vi "FPGA Main.vi"() -> ()   [LabVIEW 2017]
uses:
  Controls/Logging Settings FPGA.ctl
  Controls/Manual Control FPGA.ctl
  <vilib>/rvi/eio/common/nirviEmuTemplateMethod_errors.vi
  <vilib>/rvi/Emulation/niFpgaGetClockAttributes.vi
  <vilib>/rvi/Emulation/niFpgaSctlEmulationGetInTimedLoop.vi
  <vilib>/rvi/Emulation/niFpgaEmulationReportErrorSimple.vi
  <vilib>/rvi/Emulation/niFpgaProcessEmulError.vi
  <vilib>/rvi/interface/RandomDataEmulation/niFpgaRandomDataHandleErrors.vi
  <vilib>/rvi/Emulation/niFpgaCriticalErrorInLSC.vi
  <vilib>/eio/EIONode/EIONode.xnode
  <vilib>/rvi/DataTransferAndStorage/Container/XNode/niFpgaContainer.xnode
  <vilib>/rvi/interface/RandomDataEmulation/nirviRandomDataFpgaReadWriteTemplate.vi
panel:
  out "Emergency Triggered":bool
  in  "Emergency Normally Open/Closed":bool
  in  "Actuator Settings":T1 {"Emergency State" items=["Closed", "Open"]; "Output Port" items=["DIDO/DO0", "DIDO/DO1", "DIDO/DO2", "DIDO/DO3", "DIDO/DO4", "DIDO/DO5", "DIDO/DO6", "DIDO/DO7", "DIDO/DO8", "DIDO/DO9", "DIDO/DO10", "DIDO/DO11", "DIDO/DO12", "DIDO/DO13", "DIDO/DO14", "DIDO/DO15", "PWM/DO0", "PWM/DO1", "PWM/DO2", "PWM/DO3", "PWM/DO4", "PWM/DO5", "PWM/DO6", "PWM/DO7"]; "Unpowered State" items=["Closed", "Opened"]}
  in  "Logging Settings":T2
  out "LC FIFO Timed Out":bool
  out "PS FIFO Timed Out":bool
  in  "Poll Rate":u32
  in  "Logging?":bool
  out "TC FIFO Timed Out":bool
  in  "High Speed?":bool
  out "Automated Sequence Timer":i32
  in  "Emergency Shutdown":bool
  in  "Start Automated Sequence":bool
  in  "Manual Mode":bool=TRUE
  out "FPGA States":T3(ring)
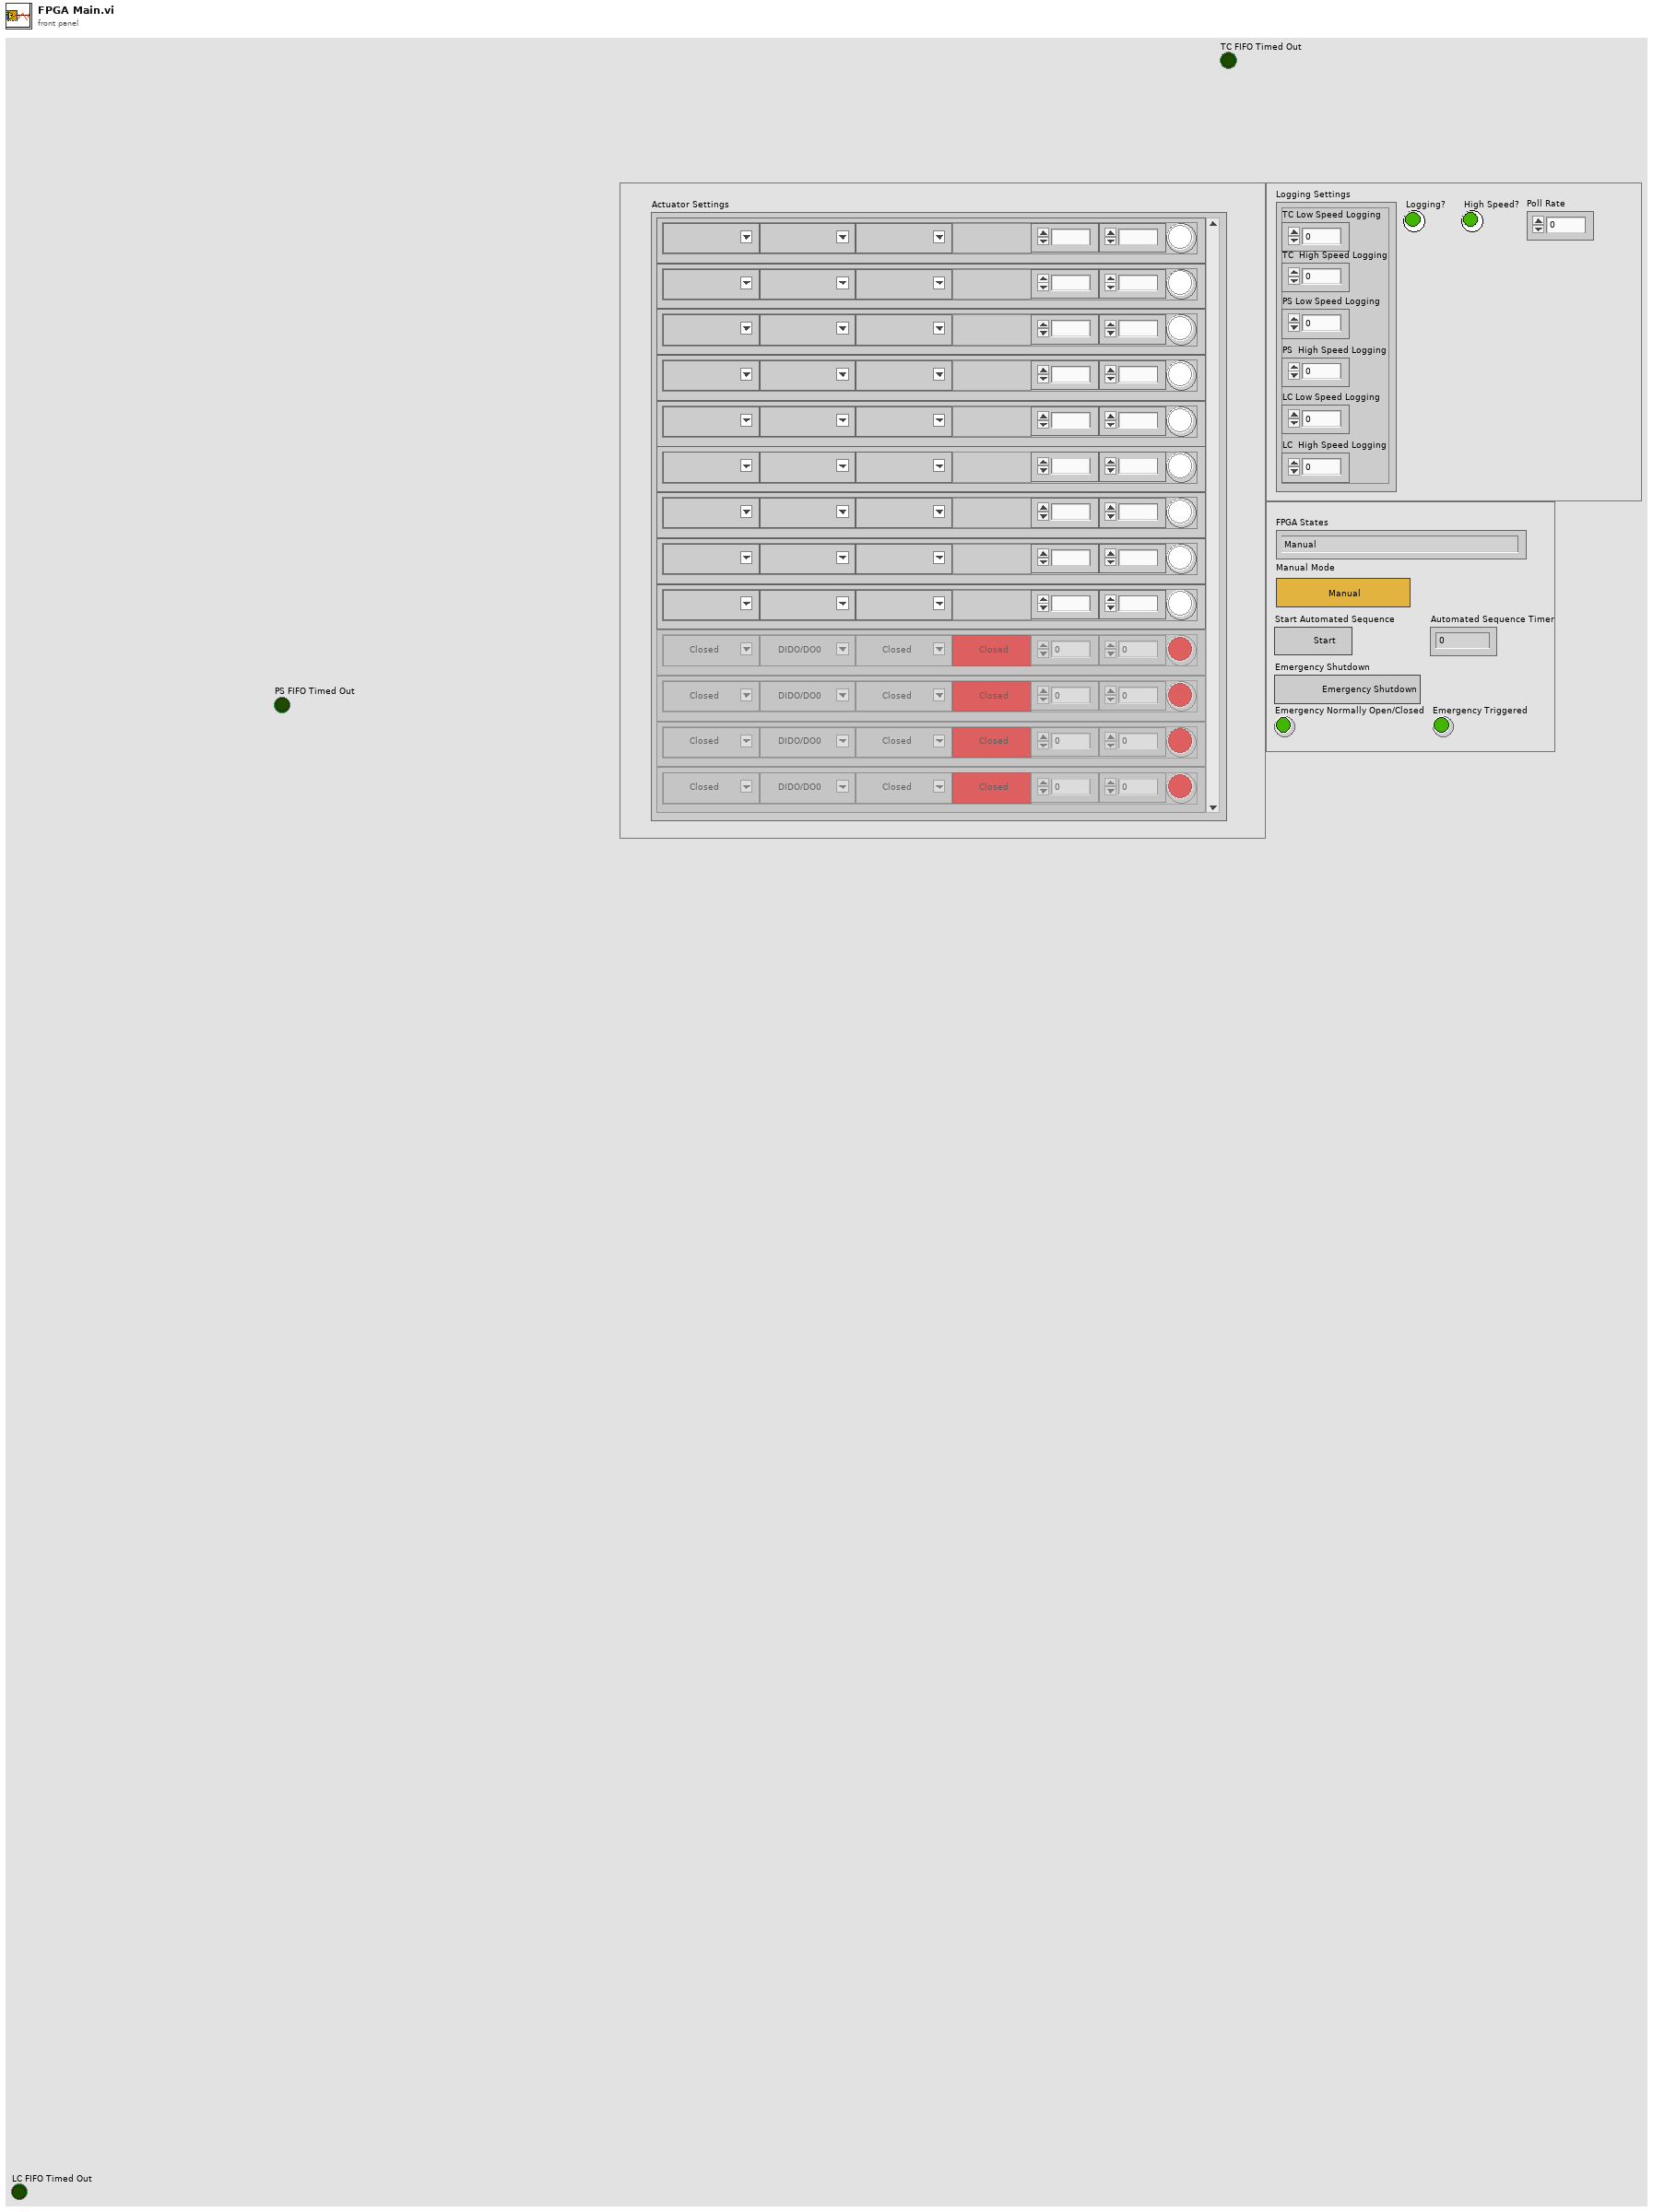
[diagram p1: front panel]
types:
  T1 = typedef "Manual Control FPGA.ctl" = cluster{"Unpowered State":u8, "Output Port":u8, "Emergency State":u8, "Blank Button":bool, "Open Time [ms]":fxp<+/-,18,18>, "Close Time [ms]":fxp<+/-,18,18>, "Active":bool}[]
  T2 = typedef "Logging Settings FPGA.ctl" = cluster{"TC Low Speed Logging":u32, "TC  High Speed Logging":u32, "PS Low Speed Logging":u32, "PS  High Speed Logging":u32, "LC Low Speed Logging":u32, "LC  High Speed Logging":u32}
  T3 = enum16{"Manual", "Standby", "Automated Sequence", "Automated Sequence End", "Emergency"}
  T4 = cluster{"Unpowered State":u8, "Output Port":u8, "Emergency State":u8, "Blank Button":bool, "Open Time [ms]":fxp<+/-,18,18>, "Close Time [ms]":fxp<+/-,18,18>, "Active":bool}
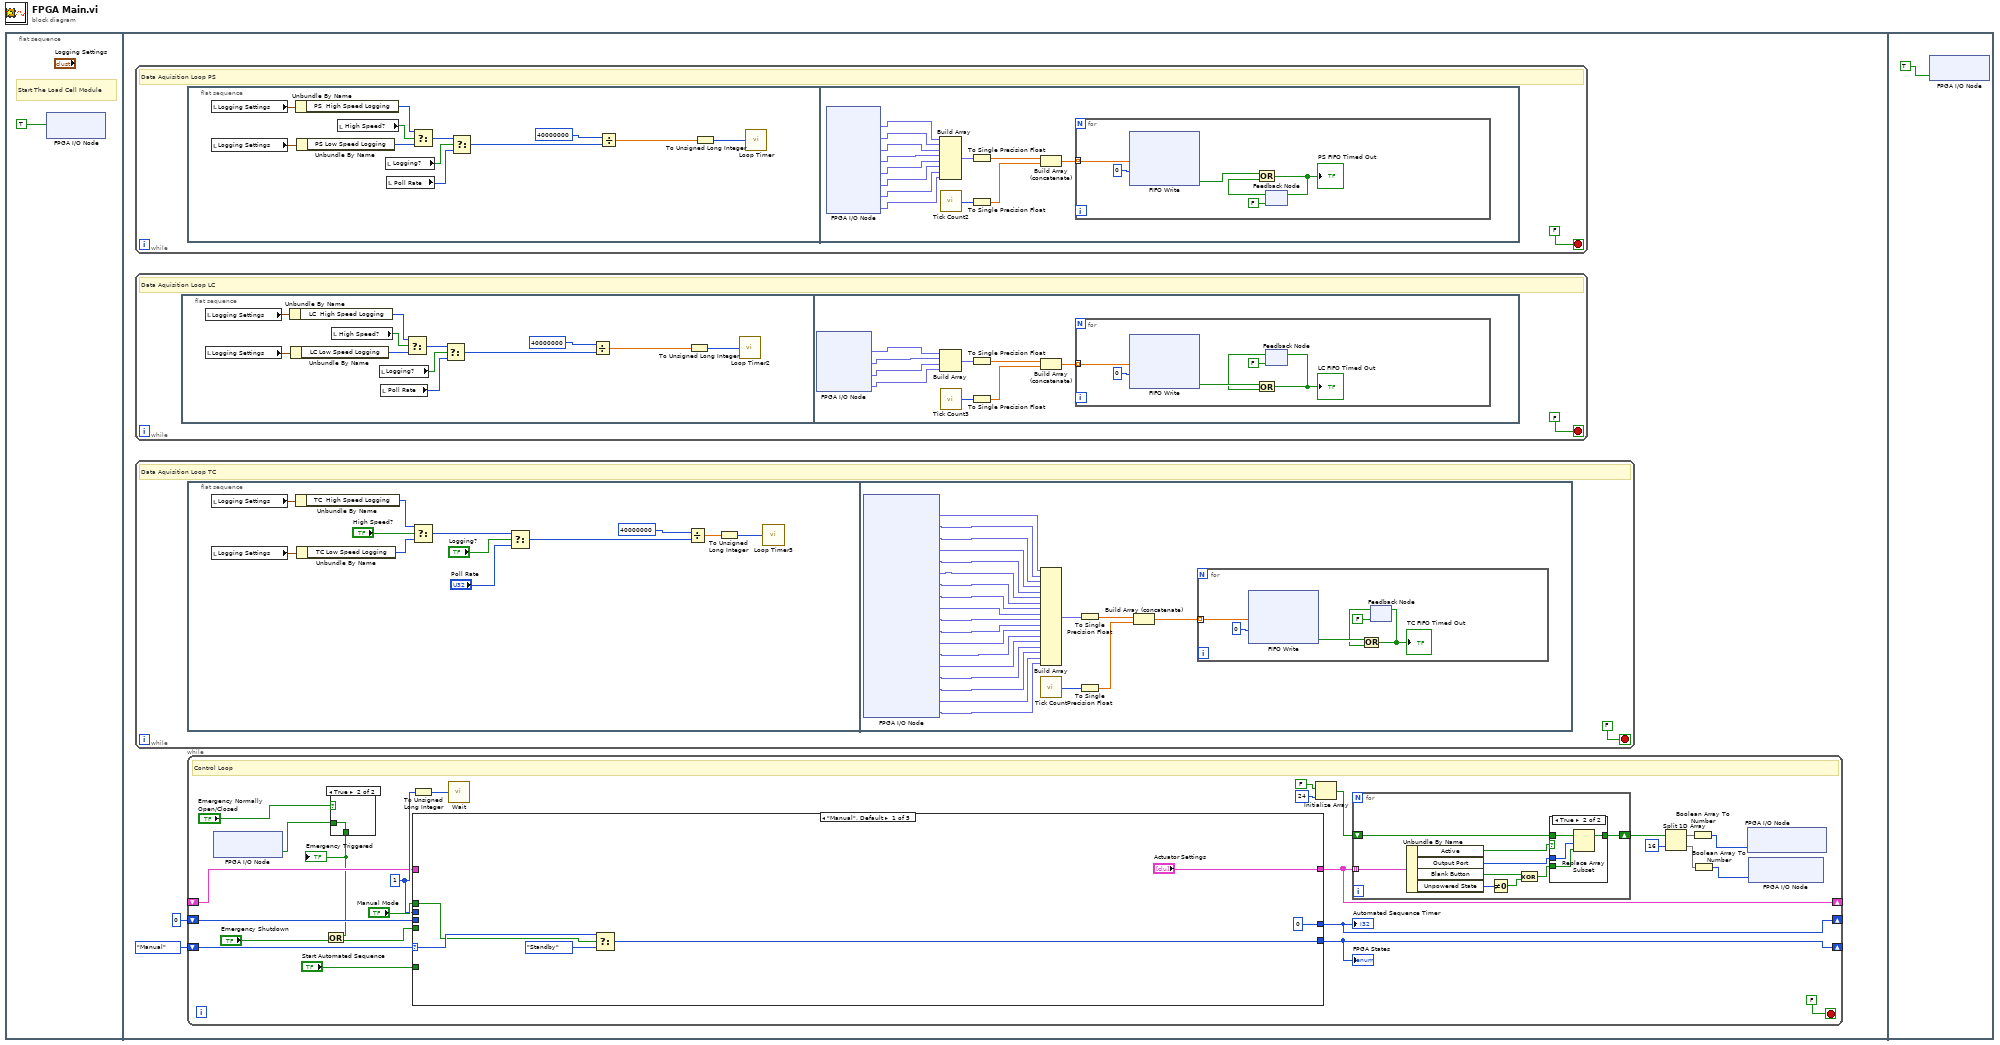
[diagram p0: block diagram]
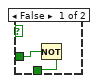
[diagram p2: hidden frame]
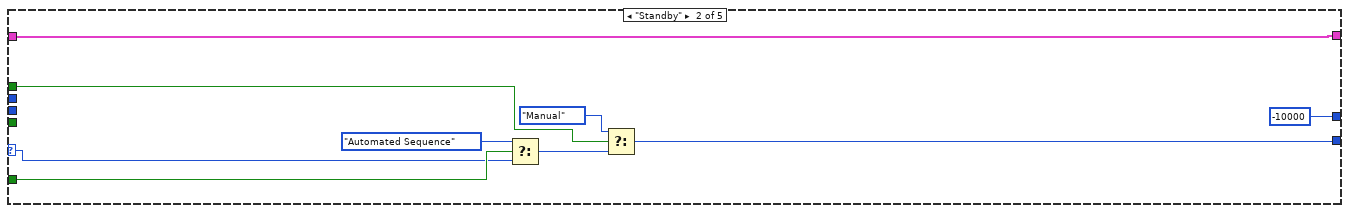
[diagram p4: hidden frame]
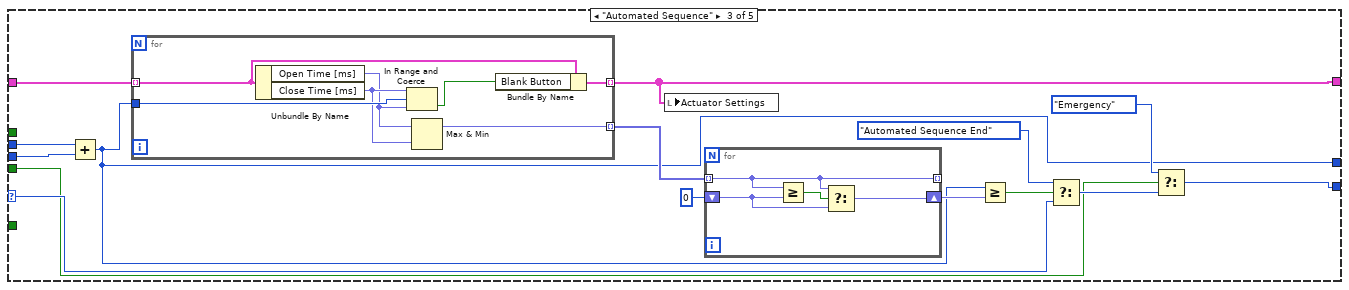
[diagram p5: hidden frame]
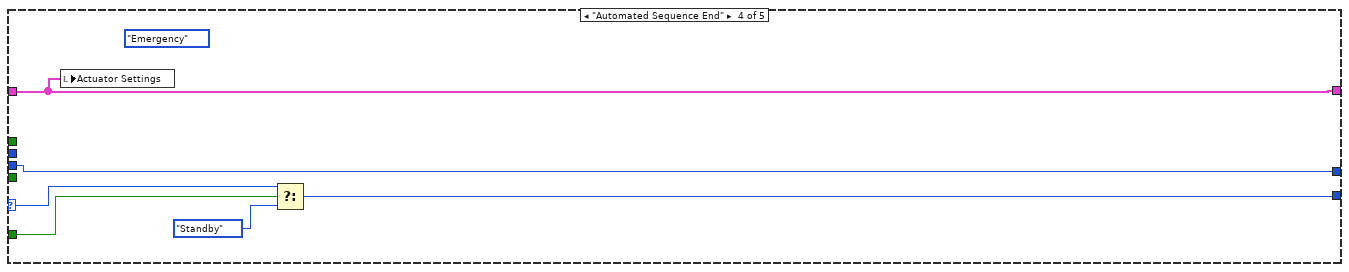
[diagram p6: hidden frame]
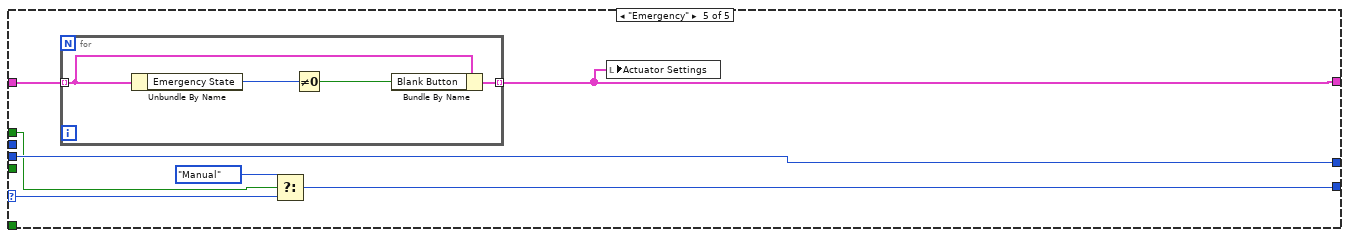
[diagram p7: hidden frame]
diagram:
  n1 = flat-sequence {
    frame #0 {
      # "Start The Load Cell Module"
      n2 = xnode "FPGA I/O Node"("LC/Start"=TRUE) -> ()  [unwired: 1 in, 1 out]
    }
    frame #1 {
      n3 = while {
        stop <- FALSE stop-if-true
        # "Data Aquisition Loop PS"
        n4 = flat-sequence {
          frame #0 {
            n5 = local read "Logging Settings"() -> (w139:T2)
            n6 = local read "Logging Settings"() -> (w137:T2)
            n7 = Unbundle By Name(w139) -> ("PS  High Speed Logging"=w134:u32)
            n8 = Unbundle By Name(w137) -> ("PS Low Speed Logging"=w133:u32)
            n9 = local read "High Speed?"() -> (w138:bool)
            n10 = local read "Logging?"() -> (w136:bool)
            n11 = local read "Poll Rate"() -> (w135:u32)
            n12 = Select(t=w134, s=w138, f=w133) -> (s? t:f=w141:u32)
            n13 = Select(t=w141, s=w136, f=w135) -> (s? t:f=w140:u32)
            n14 = Divide(x=u32 40000000, y=w140) -> (x/y=w143:sgl)
            n15 = To Unsigned Long Integer(number=w143) -> (unsigned 32bit integer=w142:u32)
            n16 = call "Loop Timer"("Count(Ticks)"=w142) -> ()  [unwired: 1 out]
          }
          frame #1 {
            n17 = xnode "FPGA I/O Node"() -> ("PS/AI0"=w152:fxp<+/-,21,-4>, "PS/AI1"=w151:fxp<+/-,21,-4>, "PS/AI2"=w150:fxp<+/-,21,-4>, "PS/AI3"=w149:fxp<+/-,21,-4>, "PS/AI4"=w148:fxp<+/-,21,-4>, "PS/AI5"=w147:fxp<+/-,21,-4>, "PS/AI6"=w146:fxp<+/-,21,-4>, "PS/AI7"=w145:fxp<+/-,21,-4>)  [unwired: 8 in, 8 out]
            n18 = Build Array(w152, w151, w150, w149, w148, w147, w146, w145) -> (w157:fxp<+/-,21,-4>[])
            n19 = call "Tick Count2"() -> ("Tick Count(uSec)"=w155:u32)
            n20 = To Single Precision Float(number=w157) -> (single precision float=w153:sgl[])
            n21 = To Single Precision Float(number=w155) -> (single precision float=w154:sgl)
            n22 = Build Array (concatenate)(w153, w154) -> (w156:sgl[])
            n23 = for {
              tunnel: w156 -> [w163] mode=indexing
              n24 = xnode ("FIFO Write")("Element"=w163, "Timeout"=0) -> ("Timed Out?"=w161:bool)  [unwired: 1 in, 1 out]
              n25 = feedback #1(FALSE ("Timed Out?")) -> (w158:bool)
              n26 = Or(x=w161, y=w158) -> (x .or. y?=w159:bool)
              "PS FIFO Timed Out" <- w159
              n27 = feedback-in #1(w159) -> ()
            }
          }
        }
      }
      n28 = while {
        stop <- FALSE stop-if-true
        # "Data Aquisition Loop LC"
        n29 = flat-sequence {
          frame #0 {
            n30 = local read "Logging Settings"() -> (w112:T2)
            n31 = local read "Logging Settings"() -> (w110:T2)
            n32 = Unbundle By Name(w112) -> ("LC  High Speed Logging"=w106:u32)
            n33 = Unbundle By Name(w110) -> ("LC Low Speed Logging"=w107:u32)
            n34 = local read "High Speed?"() -> (w111:bool)
            n35 = local read "Logging?"() -> (w109:bool)
            n36 = local read "Poll Rate"() -> (w108:u32)
            n37 = Select(t=w106, s=w111, f=w107) -> (s? t:f=w105:u32)
            n38 = Select(t=w105, s=w109, f=w108) -> (s? t:f=w113:u32)
            n39 = Divide(x=u32 40000000, y=w113) -> (x/y=w115:sgl)
            n40 = To Unsigned Long Integer(number=w115) -> (unsigned 32bit integer=w114:u32)
            n41 = call "Loop Timer2"("Count(Ticks)"=w114) -> ()  [unwired: 1 out]
          }
          frame #1 {
            n42 = xnode "FPGA I/O Node"() -> ("LC/AI0"=w120:fxp<+/-,24,-4>, "LC/AI1"=w119:fxp<+/-,24,-4>, "LC/AI2"=w118:fxp<+/-,24,-4>, "LC/AI3"=w117:fxp<+/-,24,-4>)  [unwired: 4 in, 4 out]
            n43 = Build Array(w120, w119, w118, w117) -> (w125:fxp<+/-,24,-4>[])
            n44 = call "Tick Count3"() -> ("Tick Count(uSec)"=w123:u32)
            n45 = To Single Precision Float(number=w125) -> (single precision float=w121:sgl[])
            n46 = To Single Precision Float(number=w123) -> (single precision float=w122:sgl)
            n47 = Build Array (concatenate)(w121, w122) -> (w124:sgl[])
            n48 = for {
              tunnel: w124 -> [w131] mode=indexing
              n49 = xnode ("FIFO Write")("Element"=w131, "Timeout"=0) -> ("Timed Out?"=w129:bool)  [unwired: 1 in, 1 out]
              n50 = feedback #2(FALSE ("Timed Out?")) -> (w126:bool)
              n51 = Or(x=w129, y=w126) -> (x .or. y?=w127:bool)
              "LC FIFO Timed Out" <- w127
              n52 = feedback-in #2(w127) -> ()
            }
          }
        }
      }
      n53 = while {
        stop <- FALSE stop-if-true
        # "Data Aquisition Loop TC"
        n54 = flat-sequence {
          frame #0 {
            n55 = local read "Logging Settings"() -> (w168:T2)
            n56 = local read "Logging Settings"() -> (w166:T2)
            n57 = Unbundle By Name(w168) -> ("TC  High Speed Logging"=w167:u32)
            n58 = Unbundle By Name(w166) -> ("TC Low Speed Logging"=w165:u32)
            n59 = Select(t=w167, s="High Speed?", f=w165) -> (s? t:f=w171:u32)
            n60 = Select(t=w171, s="Logging?", f="Poll Rate") -> (s? t:f=w169:u32)
            n61 = Divide(x=u32 40000000, y=w169) -> (x/y=w174:sgl)
            n62 = To Unsigned Long Integer(number=w174) -> (unsigned 32bit integer=w173:u32)
            n63 = call "Loop Timer3"("Count(Ticks)"=w173) -> ()  [unwired: 1 out]
          }
          frame #1 {
            n64 = xnode "FPGA I/O Node"() -> ("TC/TC0"=w194:fxp<+/-,24,-2>, "TC/TC1"=w193:fxp<+/-,24,-2>, "TC/TC2"=w192:fxp<+/-,24,-2>, "TC/TC3"=w191:fxp<+/-,24,-2>, "TC/TC4"=w190:fxp<+/-,24,-2>, "TC/TC5"=w177:fxp<+/-,24,-2>, "TC/TC6"=w189:fxp<+/-,24,-2>, "TC/TC7"=w188:fxp<+/-,24,-2>, "TC/TC8"=w187:fxp<+/-,24,-2>, "TC/TC9"=w186:fxp<+/-,24,-2>, "TC/TC10"=w185:fxp<+/-,24,-2>, "TC/TC11"=w184:fxp<+/-,24,-2>, "TC/TC12"=w183:fxp<+/-,24,-2>, "TC/TC13"=w182:fxp<+/-,24,-2>, "TC/TC14"=w181:fxp<+/-,24,-2>, "TC/TC15"=w180:fxp<+/-,24,-2>, "TC/Autozero"=w179:fxp<+/-,24,-2>, "TC/CJC"=w178:fxp<+/-,24,-2>)  [unwired: 18 in, 18 out]
            n65 = Build Array(w194, w193, w192, w191, w190, w177, w189, w188, w187, w186, w185, w184, w183, w182, w181, w180, w179, w178) -> (w199:fxp<+/-,24,-2>[])
            n66 = call "Tick Count"() -> ("Tick Count(uSec)"=w197:u32)
            n67 = To Single Precision Float(number=w199) -> (single precision float=w195:sgl[])
            n68 = To Single Precision Float(number=w197) -> (single precision float=w196:sgl)
            n69 = Build Array (concatenate)(w195, w196) -> (w198:sgl[])
            n70 = for {
              tunnel: w198 -> [w205] mode=indexing
              n71 = xnode ("FIFO Write")("Element"=w205, "Timeout"=0) -> ("Timed Out?"=w203:bool)  [unwired: 1 in, 1 out]
              n72 = feedback #3(FALSE ("Timed Out?")) -> (w200:bool)
              n73 = Or(x=w203, y=w200) -> (x .or. y?=w201:bool)
              "TC FIFO Timed Out" <- w201
              n74 = feedback-in #3(w201) -> ()
            }
          }
        }
      }
      n75 = while {
        shift-right: [w27] -> _
        shift-left: T3."Manual" ("FPGA States") -> [w28]
        shift-right: [w11] -> _
        shift-left: _ -> [w18]
        shift-right: [w23] -> _
        shift-left: 0 -> [w22]
        stop <- FALSE stop-if-true
        w21 = 1 ("Count(mSec)")
        # "Control Loop"
        n76 = xnode "FPGA I/O Node"() -> ("DIDO/DI15"=w6:bool)  [unwired: 1 in, 1 out]
        n77 = case shown="True" "Emergency Normally Open/Closed" {
          tunnel: w6 -> [w29 w31]
          tunnel: [w30 w31] -> w9
          frame False {
            n78 = Not(x=w29) -> (.not. x?=w30:bool)
          }
          frame True {
          }
        }
        "Emergency Triggered" <- w9
        n79 = Or(x=w9, y="Emergency Shutdown") -> (x .or. y?=w10:bool)
        n80 = To Unsigned Long Integer(number=w21) -> (unsigned 32bit integer=w20:u32)
        n81 = case shown="\"Manual\", Default" w28 {
          selector: w28 -> [w51 w59 w73 w90 w97]
          tunnel: [w48 w54 w74 w88 w95] -> w27
          tunnel: w10 -> [_ _ w70 _ _]
          tunnel: "Start Automated Sequence" -> [_ w60 _ w91 _]
          tunnel: "Manual Mode" -> [w49 w57 _ _ w98]
          tunnel: [0 -10000 w63 w92 w99] -> w23
          tunnel: w22 -> [_ _ w69 w92 w99]
          tunnel: w21 -> [_ _ w68 _ _]
          tunnel: ["Actuator Settings" w52 w62 w87 w93] -> w11
          tunnel: w18 -> [_ w52 w64 w87 w94]
          frame "Manual", Default {
            n82 = Select(t=w51, s=w49, f=T3."Standby") -> (s? t:f=w48:T3)
          }
          frame "Standby" {
            n83 = Select(t=T3."Automated Sequence", s=w60, f=w59) -> (s? t:f=w56:T3)
            n84 = Select(t=T3."Manual", s=w57, f=w56) -> (s? t:f=w54:T3)
          }
          frame "Automated Sequence" {
            n85 = Add(x=w68, y=w69) -> (x+y=w63:i32)
            n86 = for {
              tunnel: w64 -> [w77] mode=indexing
              tunnel: [w82] -> w65 mode=indexing
              tunnel: w63 -> [w81]
              tunnel: [w76] -> w62 mode=indexing
              n87 = Unbundle By Name(w77) -> ("Open Time [ms]"=w79:fxp<+/-,18,18>, "Close Time [ms]"=w80:fxp<+/-,18,18>)
              n88 = In Range and Coerce(upper limit=w80, x=w81, lower limit=w79) -> (In Range?=w78:bool)  [unwired: 1 out]
              n89 = Max & Min(x=w79, y=w80) -> (max(x,y)=w82:fxp<+/-,18,18>)  [unwired: 1 out]
              n90 = Bundle By Name(cluster=w77, "Blank Button"=w78) -> (w76:T4)
            }
            n91 = local write "Actuator Settings"(w62) -> ()
            n92 = for {
              tunnel: [w83] -> _ mode=indexing
              shift-right: [w86] -> w66
              shift-left: 0 ("y") -> [w84]
              tunnel: w65 -> [w83] mode=indexing
              n93 = Greater Or Equal?(x=w83, y=w84) -> (x >= y?=w85:bool)
              n94 = Select(t=w83, s=w85, f=w84) -> (s? t:f=w86:fxp<+/-,32,32>)
            }
            n95 = Greater Or Equal?(x=w63, y=w66) -> (x >= y?=w61:bool)
            n96 = Select(t=T3."Automated Sequence End", s=w61, f=w73) -> (s? t:f=w71:T3)
            n97 = Select(t=T3."Emergency", s=w70, f=w71) -> (s? t:f=w74:T3)
          }
          frame "Automated Sequence End" {
            (unwired) T3."Emergency" ("t")
            n98 = local write "Actuator Settings"(w87) -> ()
            n99 = Select(t=w90, s=w91, f=T3."Standby" ("FPGA States")) -> (s? t:f=w88:T3)
          }
          frame "Emergency" {
            n100 = for {
              tunnel: w94 -> [w103] mode=indexing
              tunnel: [w100] -> w93 mode=indexing
              n101 = Unbundle By Name(w103) -> ("Emergency State"=w101:u8)
              n102 = Not Equal To 0?(x=w101) -> (x != 0?=w102:bool)
              n103 = Bundle By Name(cluster=w103, "Blank Button"=w102) -> (w100:T4)
            }
            n104 = Select(t=T3."Manual", s=w98, f=w97) -> (s? t:f=w95:T3)
            n105 = local write "Actuator Settings"(w93) -> ()
          }
        }
        "FPGA States" <- w27
        "Automated Sequence Timer" <- w23
        n106 = call "Wait"("Count(mSec)"=w20) -> ()  [unwired: 1 out]
        n107 = Initialize Array(FALSE, 24 ("dimension size")) -> (w16:bool[])
        n108 = for {
          tunnel: w11 -> [w40] mode=indexing
          shift-right: [w35] -> w15
          shift-left: w16 -> [w36]
          n109 = Unbundle By Name(w40) -> ("Active"=w32:bool, "Output Port"=w34:u8, "Blank Button"=w39:bool, "Unpowered State"=w38:u8)
          n110 = Not Equal To 0?(x=w38) -> (x != 0?=w37:bool)
          n111 = Exclusive Or(1:w37, 2:w39) -> (0:w33:bool)
          n112 = case shown="True" w32 {
            tunnel: w36 -> [w41 w45]
            tunnel: [w41 w44] -> w35
            tunnel: w34 -> [_ w43]
            tunnel: w33 -> [_ w42]
            frame False {
            }
            frame True {
              n113 = Replace Array Subset(array=w45, new element=w42, index=w43) -> (w44:bool[])
            }
          }
        }
        n114 = Split 1D Array(array=w15, index=16) -> (first subarray=w13:bool[], second subarray=w5:bool[])
        n115 = Boolean Array To Number(Boolean array=w13) -> (number=w7:u16)
        n116 = Boolean Array To Number(Boolean array=w5) -> (number=w4:u8)
        n117 = xnode "FPGA I/O Node"("DIDO/DO15:0"=w7) -> ()  [unwired: 1 in, 1 out]
        n118 = xnode "FPGA I/O Node"("PWM/DO7:0"=w4) -> ()  [unwired: 1 in, 1 out]
      }
    }
    frame #2 {
      n119 = xnode "FPGA I/O Node"("LC/Stop"=TRUE ("LC/Start")) -> ()  [unwired: 1 in, 1 out]
    }
  }
